vi "DSF.Engine.Sequencer.Process Rx.vi"(8 "error in (no error)":errorcluster, 9 "engine iteration":u64, 10 "Plugins":refnum<class "DSF.Engine.Plugin.lvclass">[](array[class]), 11 "Sequencer in":refnum<class "DSF.Engine.Sequencer.lvclass">) -> (0 "error out":errorcluster, 3 "Sequencer out":refnum<class "DSF.Engine.Sequencer.lvclass">)   [LabVIEW 2017, in "DSF.Engine.lvlib" / "DSF.Engine.Sequencer.lvclass"]
uses:
  DSF.Engine.Sequencer.lvclass
  DSF.Engine.Sequencer.Timing Bundle.lvclass
  Plugin/DSF.Engine.Plugin.lvclass
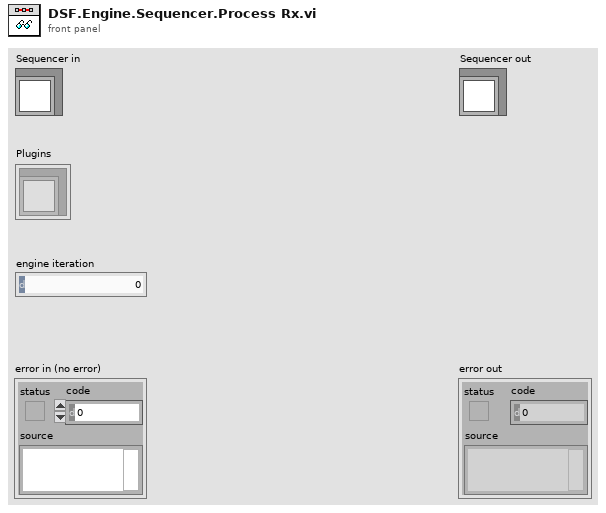
[diagram p1: front panel]
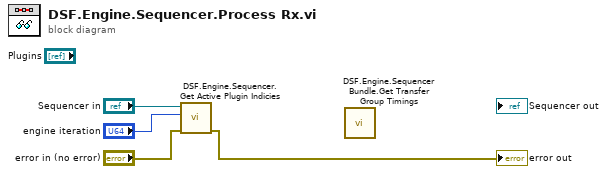
[diagram p0: block diagram]
diagram:
  n1 = call "DSF.Engine.Sequencer.Get Active Plugin Indicies.vi"("error in (no error)"="error in (no error)", "Plugins"="engine iteration", "Sequencer in"="Sequencer in") -> ("error out"=→"error out":errorcluster)  [unwired: 6 in, 2 out]
  n2 = call "DSF.Engine.Sequencer Bundle.Get Transfer Group Timings.vi"() -> ()  [unwired: 9 in, 3 out]
